vi "TaskFor_P3AT_Co_Outside_Control_Cluster_Msg.vi"(8 "error in (no error)":errorcluster caption="错误输入（无错误）", 10 "Outside_Control_Cluster":T1, 11 "Remote Endpoint P3AT输入":refnum<class "RemoteP3AT.lvclass">) -> (0 "error out":errorcluster caption="错误输出", 3 "Remote Endpoint P3AT输出":refnum<class "RemoteP3AT.lvclass">)   [LabVIEW 2014]
uses:
  RemoteP3AT.lvclass
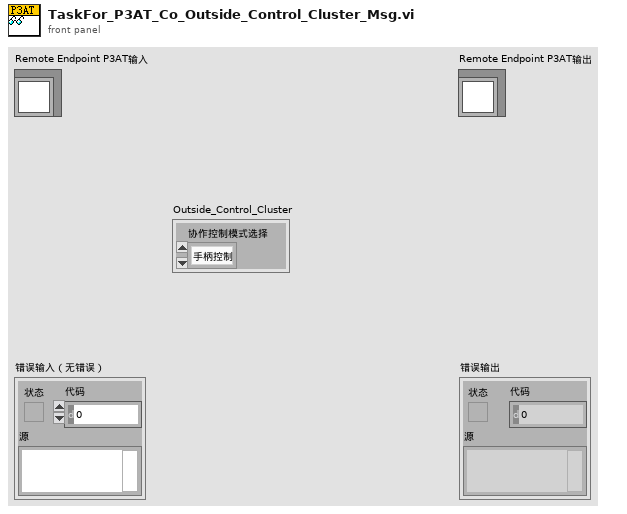
[diagram p1: front panel]
types:
  T1 = cluster{"协作控制模式选择":enum32{"手柄控制", "地图导引", "语音控制"}}
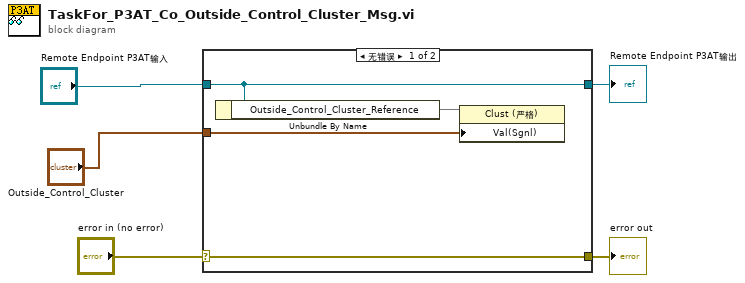
[diagram p0: block diagram]
diagram:
  n1 = case shown="无错误" "error in (no error)" {
    selector: "error in (no error)" -> [w9 w10]
    tunnel: [w9 w10] -> w4
    tunnel: [w8 w11] -> w2
    tunnel: "Remote Endpoint P3AT输入" -> [w8 w11]
    tunnel: "Outside_Control_Cluster" -> [w6 _]
    frame No Error {
      n2 = Unbundle By Name(w8) -> ("Outside_Control_Cluster_Reference"=w7)
      n3 = property class="Clust (严格)"(reference=w7, "Val(Sgnl)"=w6) -> ()  [unwired: 1 in, 2 out]
    }
    frame Error {
    }
  }
  "error out" <- w4
  "Remote Endpoint P3AT输出" <- w2
